vi "Actor Core.vi"(8 "error in":errorcluster, 11 "Time Protocol":refnum<class "Time Protocol.lvclass">) -> (0 "error out":errorcluster, 3 "Actor out":refnum<class "Actor.lvclass">)   [LabVIEW 2012, in "Time Protocol Actor.lvlib" / "Time Protocol.lvclass"]
doc: "This is Actor Core.vi, the main message handling loop for Actors. An actor usually just sits in this loop and processes messages as they arrive. Any error returned by the message Do.vi call will stop the loop, with error code 43 as the canonical signal to stop with no error sent to caller. Descendants may override that in Handle Error.vi."
uses:
  Time Protocol.lvclass
  <vilib>/ActorFramework/Actor/Actor.lvclass
  Time Protocol.lvclass/Time Protocol.ctl
  <vilib>/ActorFramework/Actor/Actor.lvclass/Actor.ctl
  <vilib>/ActorFramework/Message Enqueuer/Message Enqueuer.lvclass/Message Enqueuer.ctl
  Write Code.vi
  Write History.vi
  Write Open.vi
  Write Path.vi
  Write State.vi
  Write VI Refnum.vi
  <vilib>/ActorFramework/Message Enqueuer/Init from Existing Queue.vi
  <vilib>/ActorFramework/Message Enqueuer/Enqueue.vi
  <vilib>/ActorFramework/Message Priority Queue/Priority Enqueue.vi
  <vilib>/ActorFramework/Message Enqueuer/Message Enqueuer.lvclass
  <vilib>/ActorFramework/Stop Msg/Stop Msg.lvclass
  Time Protocol Messages/Run Protocol Msg/Run Protocol Msg.lvclass
  Time Protocol Messages/Open Protocol Msg/Open Protocol Msg.lvclass
  Time Protocol Messages/Change Status Msg/Change Status Msg.lvclass
panel:
  in  "stop signal":bool
  out "File Path Control":path
  in  "Radio Buttons":T1(radio)=enum."Media Stop Button"
  in  "Open Button":bool
  out "Code":i32(listbox)
  out "History":i32(listbox)=2
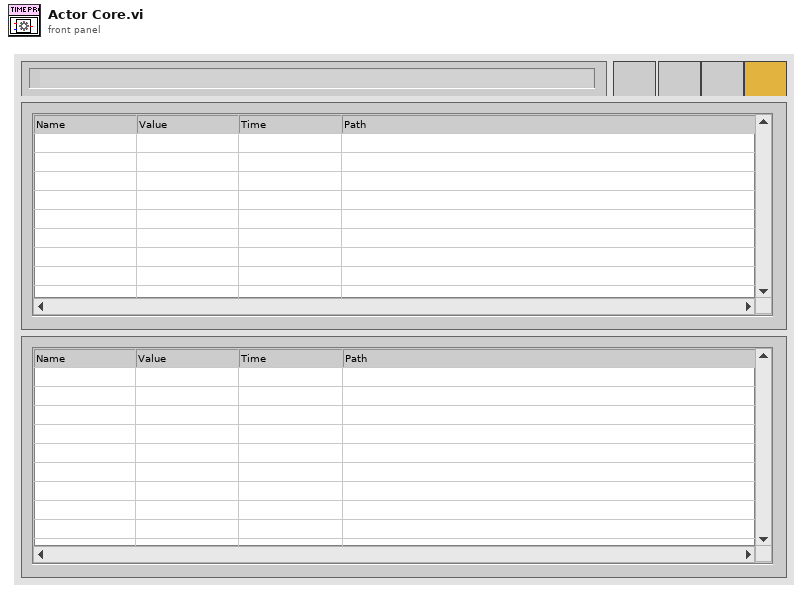
[diagram p1: front panel]
types:
  T1 = enum32{"Pause Button", "Play Button", "Media Stop Button"}
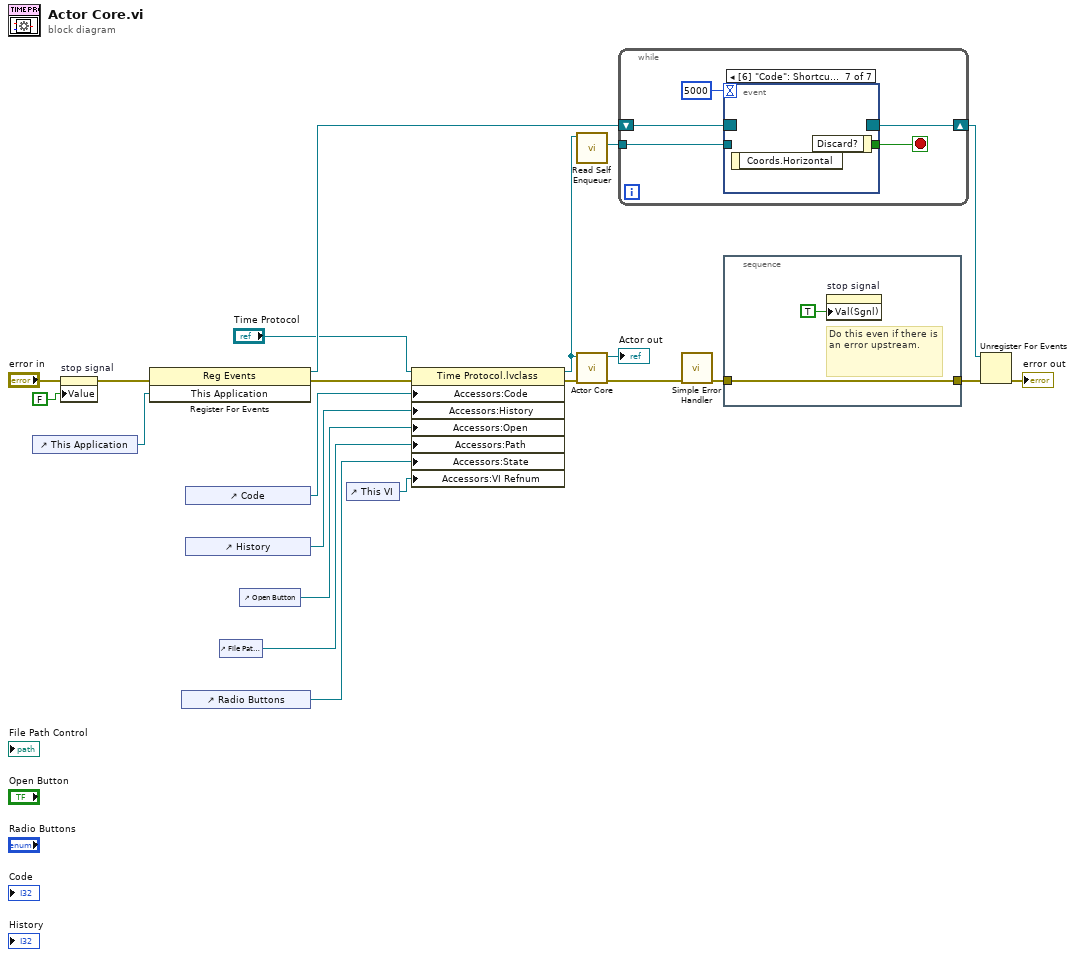
[diagram p0: block diagram]
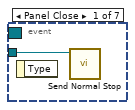
[diagram p2: hidden frame]
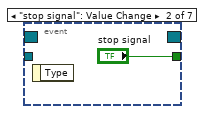
[diagram p3: hidden frame]
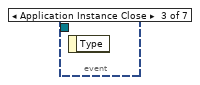
[diagram p4: hidden frame]
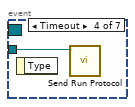
[diagram p5: hidden frame]
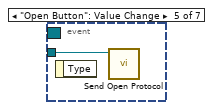
[diagram p6: hidden frame]
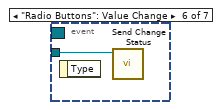
[diagram p7: hidden frame]
diagram:
  n1 = control-ref of="This Application"() -> (w14:refnum<vi>)
  n2 = property on="stop signal" class="Bool (strict)"(error in="error in", "Value"=FALSE ("stop")) -> (error out=w15:errorcluster)  [unwired: 1 in, 1 out]
  n3 = register-events(error in=w15, w14) -> (reference out=w18:refnum<event-registration>, error out=w3:errorcluster)  [unwired: 1 in]
  n4 = control-ref of="Radio Buttons"() -> (w4:refnum<vi>)
  n5 = control-ref of="Code"() -> (w8:refnum<vi>)
  n6 = control-ref of="History"() -> (w7:refnum<vi>)
  n7 = control-ref of="File Path Control"() -> (w5:refnum<vi>)
  n8 = control-ref of="Open Button"() -> (w6:refnum<vi>)
  n9 = control-ref of="This VI"() -> (w1:refnum<vi>)
  n10 = property class="Time Protocol.lvclass"(reference="Time Protocol", error in=w3, "Accessors:Code"=w8, "Accessors:History"=w7, "Accessors:Open"=w6, "Accessors:Path"=w5, "Accessors:State"=w4, "Accessors:VI Refnum"=w1) -> (reference out=w12:refnum<class "Time Protocol.lvclass">, error out=w13:errorcluster)
  n11 = call <vilib>:"Read Self Enqueuer.vi"("Actor"=w12) -> ("Self Enqueuer"=w22:refnum<class "Message Enqueuer.lvclass">)  [unwired: 10 in]
  n12 = call-parent "Actor Core.vi"("error in"=w13, "Actor in"=w12) -> ("error out"=w20:errorcluster, "Actor out"=→"Actor out":refnum<class "Actor.lvclass">)  [unwired: 8 in]
  n13 = while {
    tunnel: w22 -> [w27]
    shift-right: [w24] -> w17
    shift-left: w18 -> [w25]
    stop <- w26 stop-if-true
    n14 = event shown="[6] \"Code\": Shortcut Menu Activation?" {
      selector: w25 -> [_ _ _ _ _ _ _]
      dyn-events: [_ _ _ _ _ _ _] -> w24
      timeout: 5000 -> [_ _ _ _ _ _ _]
      tunnel: w27 -> [w28 _ _ w30 w31 w32 _]
      tunnel: [_ "stop signal" _ _ _ _ _] -> w26
      event Panel Close {
        n15 = event-data() -> ()  [unwired: 1 in, 1 out]
        n16 = call <vilib>:"Send Normal Stop.vi"("Message Enqueuer"=w28) -> ()  [unwired: 10 in, 1 out]
      }
      event "stop signal": Value Change {
        n17 = event-data() -> ()  [unwired: 1 in, 1 out]
      }
      event Application Instance Close {
        n18 = event-data() -> ()  [unwired: 1 in, 1 out]
      }
      event Timeout {
        n19 = event-data() -> ()  [unwired: 1 in, 1 out]
        n20 = call "Send Run Protocol.vi"("Message Enqueuer"=w30) -> ()  [unwired: 9 in, 2 out]
      }
      event "Open Button": Value Change {
        n21 = event-data() -> ()  [unwired: 1 in, 1 out]
        n22 = call "Send Open Protocol.vi"("Message Enqueuer"=w31) -> ()  [unwired: 9 in, 2 out]
      }
      event "Radio Buttons": Value Change {
        n23 = event-data() -> ()  [unwired: 1 in, 1 out]
        n24 = call "Send Change Status.vi"("Message Enqueuer"=w32) -> ()  [unwired: 9 in, 2 out]
      }
      event "Code": Shortcut Menu Activation? {
        n25 = event-data() -> ()  [unwired: 1 in, 1 out]
        n26 = event-data() -> ()  [unwired: 2 in, 1 out]
      }
    }
  }
  n27 = call <vilib>:"Simple Error Handler.vi"("error in (no error)"=w20) -> ("error out"=w19:errorcluster)  [unwired: 4 in, 4 out]
  n28 = stacked-sequence {
    tunnel: [w33] -> w16
    tunnel: w19 -> [w33]
    frame #0 {
      # "Do this even if there is an error upstream."
      n29 = property on="stop signal" class="Bool (strict)"("Val(Sgnl)"=TRUE ("stop")) -> ()  [unwired: 2 in, 2 out]
    }
  }
  n30 = Unregister For Events(event registration refnum=w17, error in=w16) -> (error out=→"error out":errorcluster)
